vi "Read Register.vi"(8 "error in (no error)":errorcluster, 9 "regValue":i32, 10 "regAddr":i32, 11 "_hResourceContext":u32) -> (0 "error out":errorcluster, 1 "regValue out":i32, 3 "_hResourceContext out":u32)   [LabVIEW 2013, in "QCAWLAN_DLL.lvlib"]
doc: "QCA_DLL_Export void ReadRegister(HANDLE _hResourceContext, __int32 regAddr, __int32 *regValue);"
uses:
  QCAWLAN_DLL.lvlib
  QCAWLAN_DLL.dll
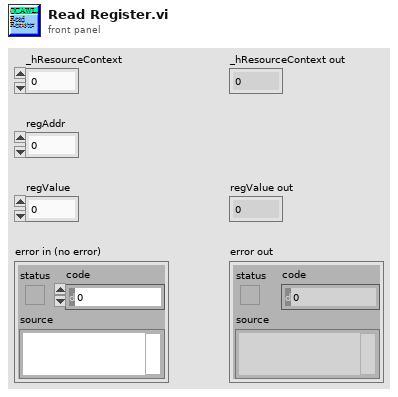
[diagram p1: front panel]
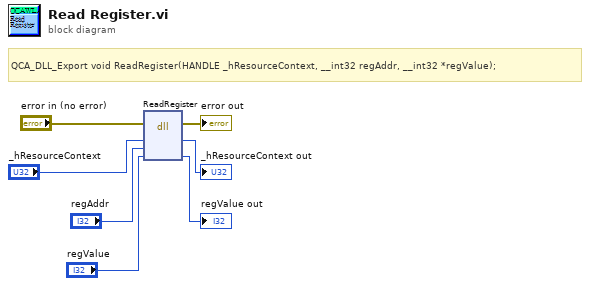
[diagram p0: block diagram]
diagram:
  # "QCA_DLL_Export void ReadRegister(HANDLE _hResourceContext, __int32 regAddr, __int32 *regValue);"
  n1 = dll-call lib="C:/Users/dave_yao/Desktop/Hitron/QCA9984 WLAN_LV2013/user.lib/QCAWLAN_DLL/QCAWLAN_DLL.*" fn="ReadRegister"(error in="error in (no error)", "_hResourceContext"="_hResourceContext", "regAddr"="regAddr", "regValue"="regValue") -> (error out=→"error out":errorcluster, "_hResourceContext"=→"_hResourceContext out":u32, "regValue"=→"regValue out":i32)  [unwired: 4 in, 1 out]
